vi "simple-move-motor.vi"() -> ()   [LabVIEW 2021]
panel:
  out "Numeric":i32
  out "pfPosition":sgl
  in  "stop":bool
  out "Motor Y\nLigado":bool=TRUE
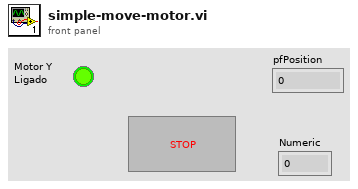
[diagram p1: front panel]
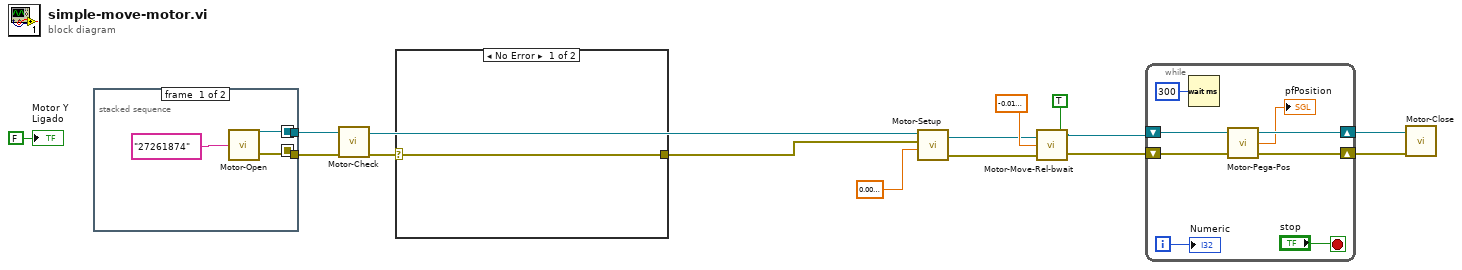
[diagram p0: block diagram]
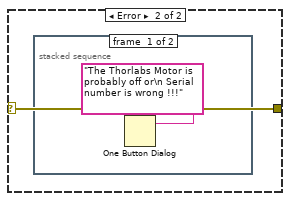
[diagram p2: hidden frame]
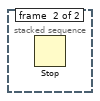
[diagram p3: hidden frame]
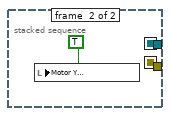
[diagram p4: hidden frame]
diagram:
  n1 = stacked-sequence {
    seq-local: [w18 _] -> [_ w21]
    seq-local: [w17 _] -> [_ w20]
    tunnel: [_ w21] -> w12
    tunnel: [_ w20] -> w11
    frame #0 {
      n2 = call "Motor-Open.vi"("S/N Motor"="27261874") -> ("MG17Motor 2"=w18:refnum<k7>, "error out"=w17:errorcluster)
    }
    frame #1 {
      n3 = local write "Motor Y\nLigado"(TRUE ("Motor3\nLigado")) -> ()
    }
  }
  n4 = call "Motor-Check.vi"("error in (no error)"=w11, "Automation Refnum in"=w12) -> ("error out"=w8:errorcluster, "Automation Refnum out"=w7:refnum<k7>)  [unwired: 8 in]
  n5 = case shown="No Error" w8 {
    selector: w8 -> [w22 w23]
    tunnel: [w22 w23] -> w6
    frame No Error {
    }
    frame Error {
      n6 = stacked-sequence {
        frame #0 {
          n7 = One Button Dialog(message="The Thorlabs Motor is probably off or\n Serial number is wrong !!!") -> ()  [unwired: 1 in, 1 out]
        }
        frame #1 {
          n8 = Stop() -> ()  [unwired: 1 in]
        }
      }
    }
  }
  n9 = call "Motor-Setup.vi"("Velocidade"=sgl 0.01, "error"=w6, "MG17Motor A"=w7) -> ("error out"=w3:errorcluster, "MG17Motor out"=w2:refnum<k7>)  [unwired: 1 in]
  n10 = call "Motor-Move-Rel-bwait.vi"("bWait"=TRUE, "error"=w3, "Posição"=sgl -0.02, "MG17Motor A"=w2) -> ("error out"=w10:errorcluster, "MG17Motor out"=w9:refnum<k7>)
  n11 = while {
    shift-right: [w30] -> w14
    shift-left: w9 -> [w32]
    shift-right: [w29] -> w13
    shift-left: w10 -> [w31]
    i -> [w25]
    stop <- "stop" stop-if-true
    n12 = Wait (ms)(milliseconds to wait=u32 300) -> ()  [unwired: 1 out]
    n13 = call "Motor-Pega-Pos.vi"("MG17Motor 2"=w32, "error out"=w31) -> ("MG17Motor 3"=w30:refnum<k7>, "pfPosition"=→"pfPosition":sgl, "error out 2"=w29:errorcluster)
    "Numeric" <- w25
  }
  n14 = call "Motor-Close.vi"("error out"=w13, "MG17Motor 3"=w14) -> ()  [unwired: 1 in]
  "Motor Y\nLigado" <- FALSE ("Motor Y\nLigado")
